vi "Result_Test.vi"(8 "error in (no error)":errorcluster caption="entrée d'erreur (pas d'erreur)", 11 "Get_Voltage en entrée":refnum<class "Pattern_Matching.lvclass">) -> (0 "error out":errorcluster caption="sortie d'erreur", 3 "Get_Voltage en sortie":refnum<class "Pattern_Matching.lvclass">)   [LabVIEW 2020, in "Library Test.lvlib" / "Pattern_Matching.lvclass"]
uses:
  Pattern_Matching.lvclass
  C:/Users/ngarcin/OneDrive - Altyor/Standard TB/Class/Test/Test (Default)/Test (Default).lvclass
  Test_Wtih_Instr/Test_With_Inst.lvclass
  Pattern_Matching.lvclass/Pattern_Matching.ctl
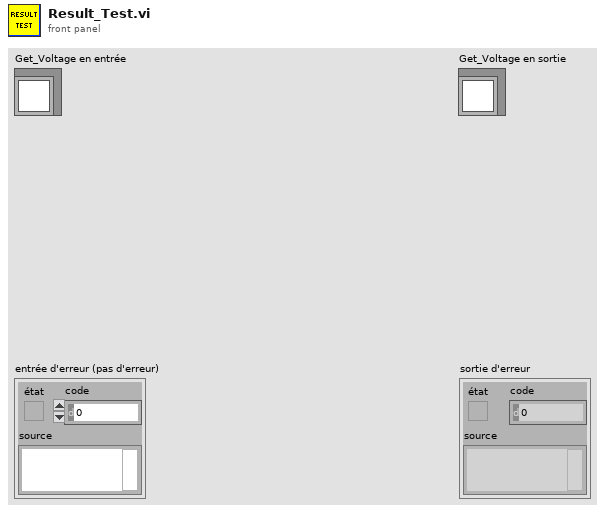
[diagram p1: front panel]
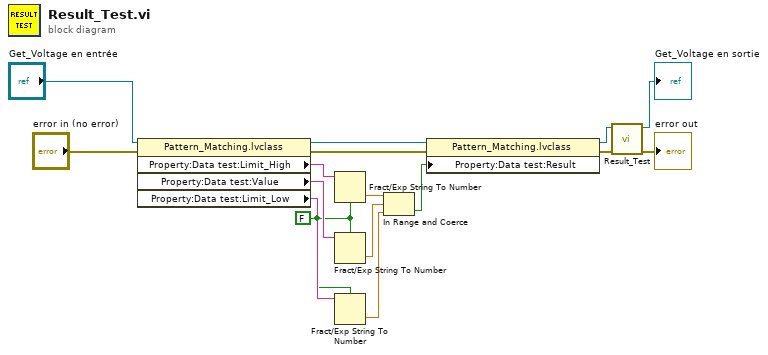
[diagram p0: block diagram]
diagram:
  w1 = FALSE ("utiliser le séparateur décimal du système (V)")
  n1 = property class="Pattern_Matching.lvclass"(reference="Get_Voltage en entrée", error in="error in (no error)") -> (reference out=w10:refnum<class "Pattern_Matching.lvclass">, error out=w8:errorcluster, "Property:Data test:Limit_High"=w16:string, "Property:Data test:Value"=w15:string, "Property:Data test:Limit_Low"=w14:string)
  n2 = Fract/Exp String To Number(use system decimal point (T)=w1, string=w16) -> (number=w13:dbl)  [unwired: 2 in, 1 out]
  n3 = Fract/Exp String To Number(use system decimal point (T)=w1, string=w15) -> (number=w12:dbl)  [unwired: 2 in, 1 out]
  n4 = Fract/Exp String To Number(use system decimal point (T)=w1, string=w14) -> (number=w11:dbl)  [unwired: 2 in, 1 out]
  n5 = In Range and Coerce(upper limit=w13, x=w12, lower limit=w11) -> (In Range?=w9:bool)  [unwired: 1 out]
  n6 = property class="Pattern_Matching.lvclass"(reference=w10, error in=w8, "Property:Data test:Result"=w9) -> (reference out=w2:refnum<class "Pattern_Matching.lvclass">, error out=w5:errorcluster)
  n7 = call-parent "Result_Test.vi"("error in (no error)"=w5, "Test_With_Inst en entrée"=w2) -> ("error out"=→"error out":errorcluster, "Test_With_Inst en sortie"=→"Get_Voltage en sortie":refnum<class "Pattern_Matching.lvclass">)  [unwired: 8 in]
